vi "Get JSON.vi"(8 "error in (no error)":errorcluster, 11 "SLSC Session In":refnum<class "SLSC Interface.lvclass">) -> (0 "error out":errorcluster, 2 "capabilities":string, 3 "SLSC Session Out":refnum<class "SLSC Interface.lvclass">)   [LabVIEW 2016, in "SLSC Switch.lvlib" / "SLSC Switch.lvclass"]
uses:
  SLSC Switch.lvclass
  <vilib>/National Instruments/SLSC Local or Remote Interface/SLSC Interface Class/SLSC Interface.lvclass
  <vilib>/National Instruments/SLSC Local or Remote Interface/SLSC Interface Class/Session Property Node/NISE.Read Dev.VendorName.vi
  <vilib>/National Instruments/SLSC Local or Remote Interface/SLSC Interface Class/Session Property Node/NISE.Read Dev.ProductNum.vi
  <vilib>/National Instruments/SLSC Local or Remote Interface/SLSC Interface Class/Session Property Node/NISE.Read Dev.SerialNum.vi
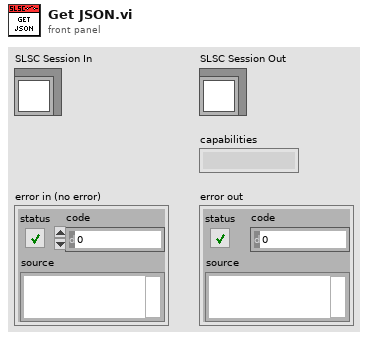
[diagram p1: front panel]
types:
  T1 = enum16{"open", "replace", "create", "open or create", "replace or create", "replace or create with confirmation"}
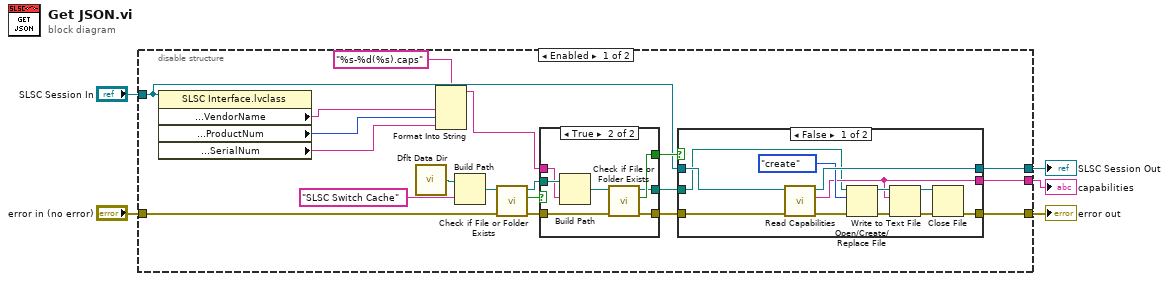
[diagram p0: block diagram]
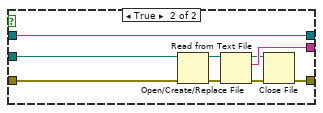
[diagram p2: hidden frame]
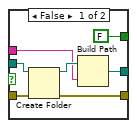
[diagram p3: hidden frame]
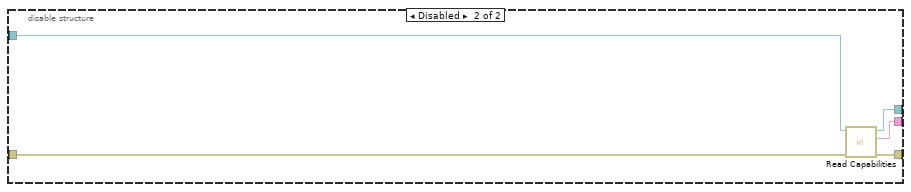
[diagram p4: hidden frame]
diagram:
  n1 = disable-structure shown="Enabled" {
    disable-tunnel: [w24 w61] -> w5
    disable-tunnel: [w21 w62] -> w4
    disable-tunnel: [w20 w63] -> w3
    disable-tunnel: "SLSC Session In" -> [w11 w64]
    disable-tunnel: "error in (no error)" -> [w13 w60]
    frame Enabled {
      n2 = property class="SLSC Interface.lvclass"(reference=w11) -> ("API:session property node:Device:Identification:Dev.VendorName"=w9:string, "API:session property node:Device:Identification:Dev.ProductNum"=w8:u32, "API:session property node:Device:Identification:Dev.SerialNum"=w7:string)  [unwired: 1 in, 2 out]
      n3 = call <vilib>:"Dflt Data Dir.vi"() -> ("App:Default Data Directory"=w15:path)
      n4 = Format Into String(format string="%s-%d(%s).caps", w9, w8, w7) -> (resulting string=w6:string)  [unwired: 2 in, 1 out]
      n5 = Build Path(base path=w15, name or relative path="SLSC Switch Cache") -> (appended path=w17:path)
      n6 = call <vilib>:"Check if File or Folder Exists.vi"("error in (no error)"=w13, "path"=w17) -> ("error out"=w14:errorcluster, "file or folder exists?"=w12:bool, "dup path"=w18:path)  [unwired: 7 in]
      n7 = case shown="True" w12 {
        tunnel: w14 -> [w51 w57]
        tunnel: w18 -> [w52 w58]
        tunnel: [FALSE ("file or folder exists?") w56] -> w19
        tunnel: [w48 w55] -> w23
        tunnel: w6 -> [w49 w54]
        tunnel: [w46 w53] -> w22
        frame False {
          n8 = Create Folder(path (use dialog)=w52, error in=w51) -> (created path=w50:path, error out=w46:errorcluster)  [unwired: 1 in, 1 out]
          n9 = Build Path(base path=w50, name or relative path=w49) -> (appended path=w48:path)
        }
        frame True {
          n10 = Build Path(base path=w58, name or relative path=w54) -> (appended path=w59:path)
          n11 = call <vilib>:"Check if File or Folder Exists.vi"("error in (no error)"=w57, "path"=w59) -> ("error out"=w53:errorcluster, "file or folder exists?"=w56:bool, "dup path"=w55:path)  [unwired: 7 in]
        }
      }
      n12 = case shown="False" w19 {
        tunnel: w22 -> [w36 w41]
        tunnel: [w25 w39] -> w24
        tunnel: w11 -> [w35 w44]
        tunnel: [w34 w44] -> w20
        tunnel: [w30 w45] -> w21
        tunnel: w23 -> [w29 w37]
        frame False {
          n13 = call "Read Capabilities.vi"("error in (no error)"=w36, "SLSC NVMEM Session In"=w35) -> ("error out"=w26:errorcluster, "capabilities"=w30:string, "SLSC NVMEM Session Out"=w34:refnum<class "SLSC Interface.lvclass">)  [unwired: 7 in]
          n14 = Open/Create/Replace File(file path (use dialog)=w29, error in=w26, operation (0:open)=T1."create") -> (refnum out=w31:refnum<file>, error out=w32:errorcluster)  [unwired: 3 in, 1 out]
          n15 = Write to Text File(file (use dialog)=w31, text=w30, error in=w32) -> (refnum out=w27:refnum<file>, error out=w28:errorcluster)  [unwired: 1 in, 1 out]
          n16 = Close File(refnum=w27, error in=w28) -> (error out=w25:errorcluster)  [unwired: 1 out]
        }
        frame True {
          n17 = Open/Create/Replace File(file path (use dialog)=w37, error in=w41) -> (refnum out=w42:refnum<file>, error out=w43:errorcluster)  [unwired: 4 in, 1 out]
          n18 = Read from Text File(file (use dialog)=w42, error in=w43) -> (refnum out=w38:refnum<file>, text=w45:string, error out=w40:errorcluster)  [unwired: 2 in, 1 out]
          n19 = Close File(refnum=w38, error in=w40) -> (error out=w39:errorcluster)  [unwired: 1 out]
        }
      }
    }
    frame Disabled {
      n20 = call "Read Capabilities.vi"("error in (no error)"=w60, "SLSC NVMEM Session In"=w64) -> ("error out"=w61:errorcluster, "capabilities"=w62:string, "SLSC NVMEM Session Out"=w63:refnum<class "SLSC Interface.lvclass">)  [unwired: 7 in]
    }
  }
  "error out" <- w5
  "capabilities" <- w4
  "SLSC Session Out" <- w3
